vi "AddTestMethod_CreateNewWizard_Invoke.vi"(10 "Cluster":T1, 11 "Wizard":T2) -> (3 "Canceled":bool)   [LabVIEW 2013]
uses:
  <resource>/Framework/Providers/API/ItemRef.ctl
  <resource>/Framework/Providers/API/mxLvNIIM.ctl
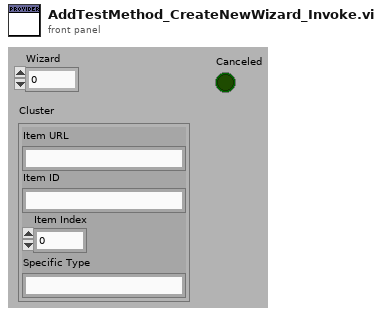
[diagram p1: front panel]
types:
  T1 = typedef "mxLvNIIM.ctl" = cluster{"Item URL":string, "Item ID":string, "Item Index":i32, "Specific Type":string}
  T2 = typedef "ItemRef.ctl" = u64
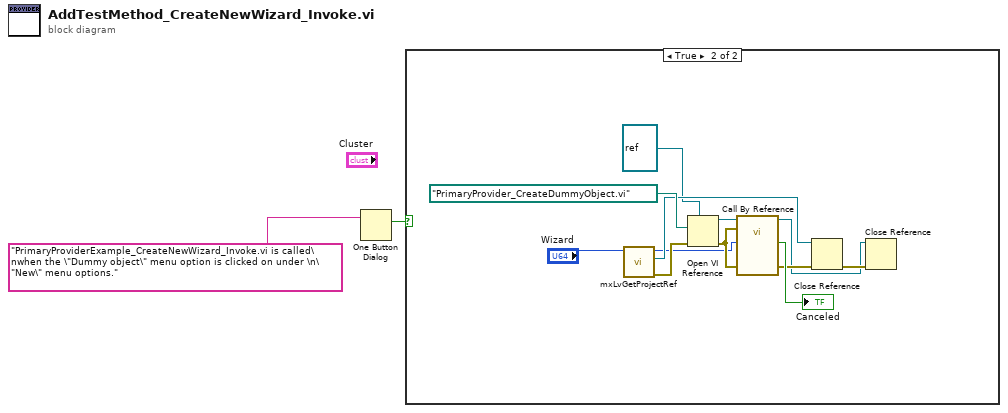
[diagram p0: block diagram]
diagram:
  n1 = One Button Dialog(message="PrimaryProviderExample_CreateNewWizard_Invoke.vi is called\nwhen the \"Dummy object\" menu option is clicked on under \n\"New\" menu options.") -> (true=w1:bool)  [unwired: 1 in]
  n2 = case shown="True" w1 {
    frame False {
    }
    frame True {
      n3 = call <resource>:"mxLvGetProjectRef.vi"("Item"="Wizard") -> ("error out"=w12:errorcluster, "Project Refnum"=w10:refnum<vi>, "Item"=w3:T2)  [unwired: 8 in]
      n4 = Open VI Reference(type specifier VI Refnum (for type only)=refnum<vi> refnum, vi path=path "PrimaryProvider_CreateDummyObject.vi", error in (no error)=w12) -> (vi reference=w5:refnum<vi>, error out=w11:errorcluster)  [unwired: 3 in]
      n5 = call-by-ref "?"(reference=w5, error in=w11, 6:"error in (no error)"=w11, "Wizard"=w3) -> (reference out=w4:refnum<vi>, "error out"=w7:errorcluster, "Cancelled?"=→"Canceled":bool)  [unwired: 6 in, 1 out]
      n6 = Close Reference(reference=w10, error in (no error)=w7) -> (error out=w9:errorcluster)
      n7 = Close Reference(reference=w4, error in (no error)=w9) -> ()  [unwired: 1 out]
    }
  }
